vi "Cmd.SwichMode.vi"(6 "Timeout [ms] (1000)":i32=1000, 7 "RunMode":T1, 8 "error in":errorcluster, 11 "cID in":refnum<k5>) -> (0 "error out":errorcluster, 3 "cID out":refnum<k5>)   [LabVIEW 2016]
uses:
  controls/RunMode.ctl
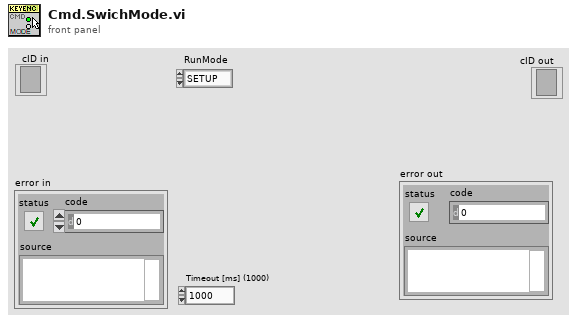
[diagram p1: front panel]
types:
  T1 = typedef "RunMode.ctl" = enum16{"SETUP", "RUN"}
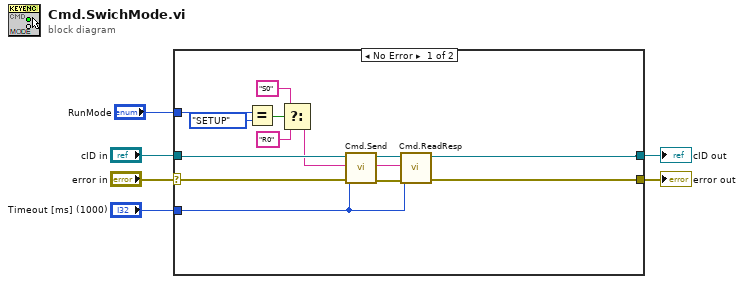
[diagram p0: block diagram]
diagram:
  n1 = case shown="No Error" "error in" {
    selector: "error in" -> [w18 w20]
    tunnel: "Timeout [ms] (1000)" -> [w15 _]
    tunnel: "cID in" -> [w19 w21]
    tunnel: [w14 w21] -> w3
    tunnel: [w13 w20] -> w2
    tunnel: "RunMode" -> [w12 _]
    frame No Error {
      n2 = Equal?(x=w12, y=RunMode."SETUP") -> (x = y?=w10:bool)
      n3 = Select(t="S0" ("format string"), s=w10, f="R0" ("format string")) -> (s? t:f=w7:string)
      n4 = call "Cmd.Send.vi"("error in (no error)"=w18, "Timeout [ms] (1000)"=w15, "Command"=w7, "connection ID"=w19) -> ("error out"=w16:errorcluster, "connection ID out"=w17:refnum<k5>)  [unwired: 6 in]
      n5 = call "Cmd.ReadResp.vi"("error in (no error)"=w16, "Timeout [ms] (1000)"=w15, "Request"=w7, "connection ID"=w17) -> ("error out"=w13:errorcluster, "connection ID out"=w14:refnum<k5>)  [unwired: 5 in, 1 out]
    }
    frame Error {
    }
  }
  "cID out" <- w3
  "error out" <- w2
